vi "Instr_InitObject.vi"(8 "error in (no error)":errorcluster, 9 "Instrument Configuration":variant, 10 "Instrument address":refnum<visa-resource-name>, 11 "Switching in":refnum<class "Switching.lvclass">) -> (0 "error out":errorcluster, 3 "Switching out":refnum<class "Switching.lvclass">)   [LabVIEW 2019, in "Switching.lvclass"]
uses:
  Switching.lvclass
  InstrControl.lvclass
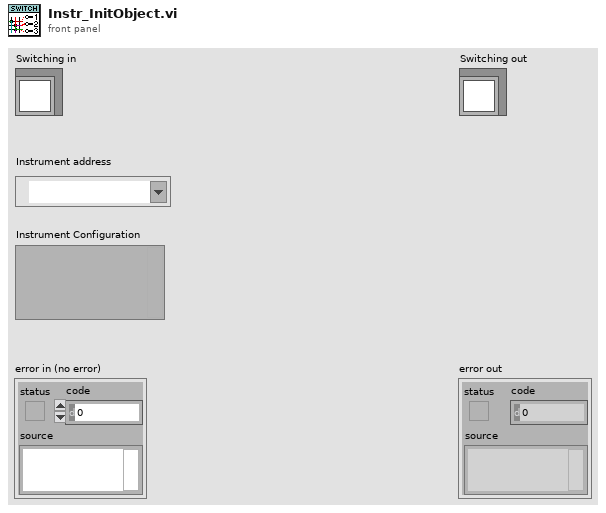
[diagram p1: front panel]
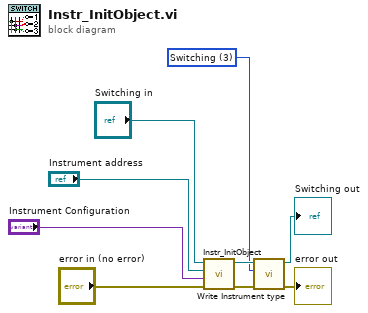
[diagram p0: block diagram]
diagram:
  w1 = u16 3 items=["Supply", "LCR", "Multimeter", "Switching"] ("Instrument type")
  n1 = call-parent "Instr_InitObject.vi"("error in (no error)"="error in (no error)", "Instrument Configuration"="Instrument Configuration", "Instrument address"="Instrument address", "InstrControl in"="Switching in") -> ("error out"=w8:errorcluster, "InstrControl out"=w7:refnum<class "Switching.lvclass">)  [unwired: 6 in]
  n2 = call-dynamic "Write Instrument type.vi"("error in (no error)"=w8, "Instrument type"=w1, "InstControl in"=w7) -> ("error out"=→"error out":errorcluster, "InstControl out"=→"Switching out":refnum<class "Switching.lvclass">)  [unwired: 7 in]
